vi "Process_GetData.vi"(0 "ref in":T3, 11 "error in":errorcluster) -> (4 "ref out":T3, 6 "Ready":bool, 8 "Mode":T2, 10 "Function":T1, 14 "Data out":T4, 15 "error out":errorcluster)   [LabVIEW 2015]
uses:
  Control/Process_Data.ctl
  Control/Process_Mode.ctl
  Control/Process_Function.ctl
  Control/Process_ref.ctl
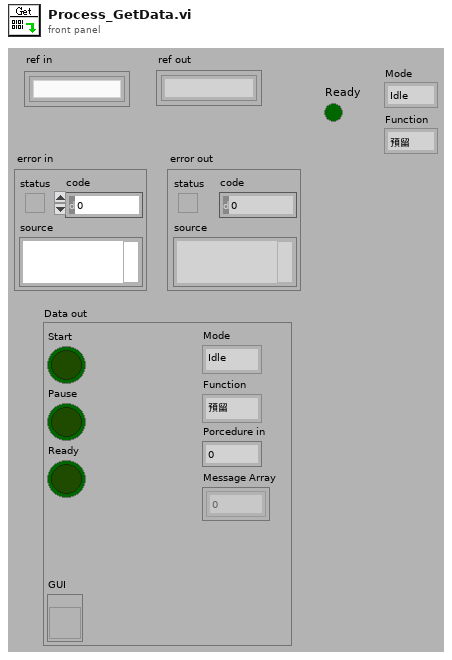
[diagram p1: front panel]
types:
  T1 = typedef "Process_Function.ctl" = enum8{"預留"}
  T2 = typedef "Process_Mode.ctl" = enum8{"Idle", "Run", "Pause", "Err"}
  T3 = typedef "Process_ref.ctl" = refnum<k1>
  T4 = typedef "Process_Data.ctl" = cluster{"GUI":refnum<vi>, "Ready":bool, "Mode":T2, "Function":T1, "Porcedure in":u8, "Message Array":i32[], "Start":bool, "Pause":bool}
  T5 = enum16{"OpenReference", "CloseReference", "Get Data", "Set Data", "Set Flag"}
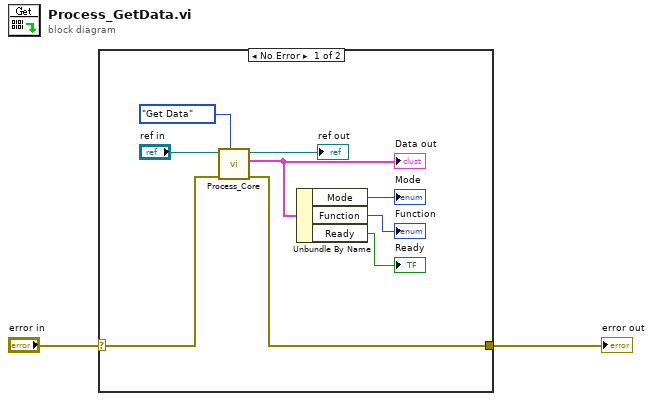
[diagram p0: block diagram]
diagram:
  n1 = case shown="No Error" "error in" {
    selector: "error in" -> [w11 w12]
    tunnel: [w10 w12] -> w1
    frame No Error {
      n2 = call "Process_Core.vi"("Function"=T5."Get Data", "error in"=w11, "ref in"="ref in") -> ("error out"=w10:errorcluster, "Data out"=w9:T4, "ref out"=→"ref out":T3)  [unwired: 5 in, 1 out]
      "Data out" <- w9
      n3 = Unbundle By Name(w9) -> ("Mode"=→"Mode":T2, "Function"=→"Function":T1, "Ready"=→"Ready":bool)
    }
    frame Error {
    }
  }
  "error out" <- w1
